vi "Get Installed Set 1.0.vi"(8 "error in (no error)":errorcluster, 10 "Cached (F)":bool, 11 "Session in":refnum<k21>) -> (0 "error out":errorcluster, 2 "Software Set":T1, 3 "Session out":refnum<k21>)   [LabVIEW 2014, in "nisyscfg.lvlib"]
uses:
  nisyscfg.lvlib
  Software Set.ctl
  Software.ctl
  Component Types.ctl
  Get Installed Set.vi
panel:
  # "This cluster is deprecated.\nUse Software Set 1.2.ctl."
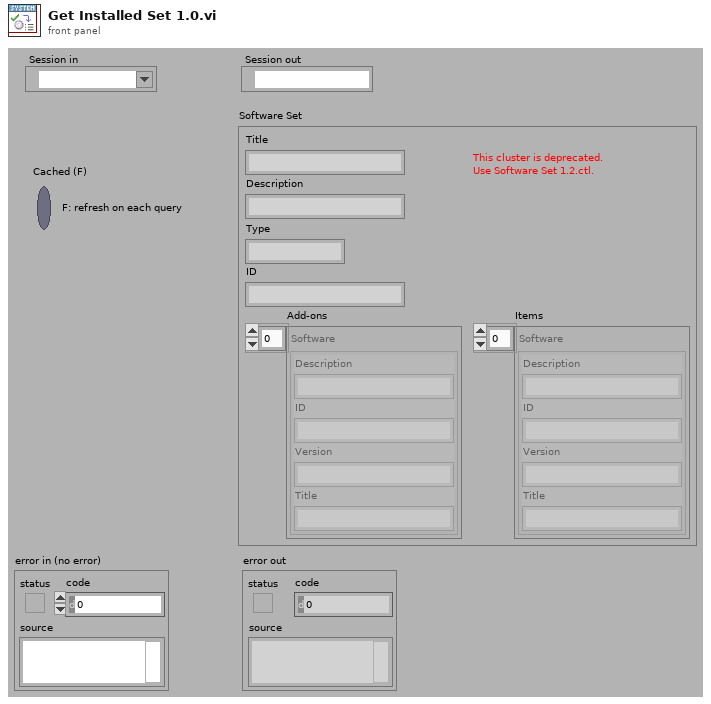
[diagram p1: front panel]
types:
  T1 = typedef "nisyscfg.lvlib/Software Set.ctl" = cluster{"Description":string, "ID":string, "Type":string, "Title":string, "Add-ons":T2[], "Items":T2[]}
  T2 = typedef "nisyscfg.lvlib/Software.ctl" = cluster{"Description":string, "ID":string, "Version":string, "Title":string}
  T3 = typedef "nisyscfg.lvlib/Component Types.ctl" = u32
  T4 = typedef "nisyscfg.lvlib/Software Set 1.2.ctl" = cluster{"information":T5, "items":T5[], "add-ons":T5[]}
  T5 = typedef "nisyscfg.lvlib/Software 1.2.ctl" = cluster{"title":string, "description":string, "ID":string, "version":string, "component type":T6}
  T6 = typedef "nisyscfg.lvlib/Component Type.ctl" = u32
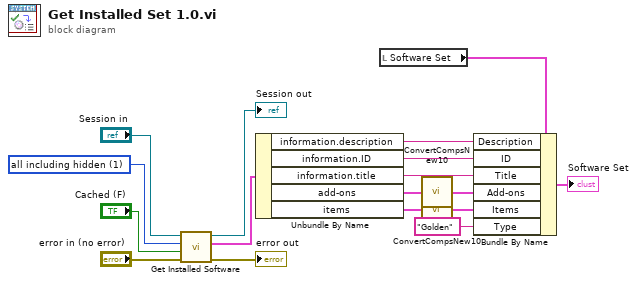
[diagram p0: block diagram]
diagram:
  w4 = T3 1 items=["all visible", "all including hidden"] ("item types (visible)")
  n1 = call-poly "Get Installed Software.vi"("error in (no error)"="error in (no error)", "Cached (F)"="Cached (F)", "Item Types (all visible)"=w4, "Session in"="Session in") -> ("error out"=→"error out":errorcluster, "Software Set"=w1:T4, "Session out"=→"Session out":refnum<k21>)  [unwired: 5 in]
  n2 = Unbundle By Name(w1) -> ("information.description"=w10:string, "information.ID"=w11:string, "information.title"=w12:string, "add-ons"=w17:T5[], "items"=w16:T5[])
  n3 = local read "Software Set"() -> (w9:T1)
  n4 = call "ConvertCompsNew10.vi"("components 1.2"=w17) -> ("components 1.0"=w13:T2[])
  n5 = call "ConvertCompsNew10.vi"("components 1.2"=w16) -> ("components 1.0"=w14:T2[])
  n6 = Bundle By Name(cluster=w9, "Description"=w10, "ID"=w11, "Title"=w12, "Add-ons"=w13, "Items"=w14, "Type"="Golden") -> (→"Software Set":T1)
